vi "GD_Infos_Auswerten.vi"(11 "Sprachliste":string[][](array[string])) -> (1 "GD Info Text":string, 2 "GD Infos Array":string[](array[string]), 3 "GD Error occured":bool)   [LabVIEW 2020, in "Linearisierung v2.lvlib" / "SpanEinstellungen.lvlib"]
uses:
  SpanEinstellungen.lvlib
  Aktion FGV GD Errors sammeln.ctl
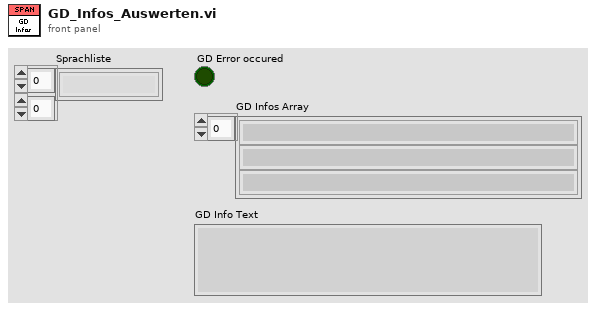
[diagram p1: front panel]
types:
  T1 = typedef "Linearisierung v2.lvlib/SpanEinstellungen.lvlib/Aktion FGV GD Errors sammeln.ctl" = enum16{"lesen", "init", "GD Infos sammeln", "Kalibrierinfos sammeln", "Test Data", "GD Infos selektiv sammeln"}
  T2 = typedef "Linearisierung v2.lvlib/SpanEinstellungen.lvlib/GD Info Cluster.ctl" = cluster{"Wobei":string, "Status":string, "Errors":T3, "Empfangsdaten":string[], "Zeitstempel":string}
  T3 = typedef "Linearisierung v2.lvlib/LIN ErrorCluster.ctl" = cluster{"Störung Kommunikation":bool, "Pressure carrier gas":bool, "Pressure diluted gas":bool, "Outlet Pressure":bool, "SNOX before SAIR":bool, "Störung Gasteiler":bool}
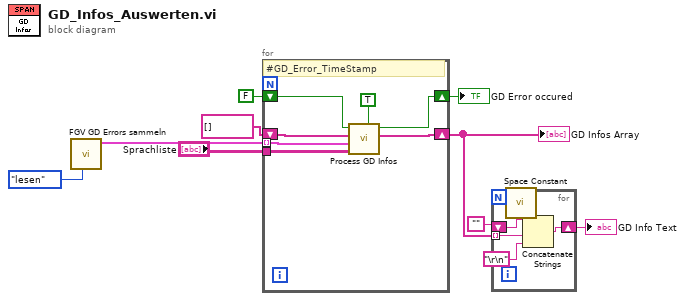
[diagram p0: block diagram]
diagram:
  n1 = call "FGV GD Errors sammeln.vi"("Aktion"=Aktion_FGV_GD_Errors_sammeln."lesen") -> ("GD Info-Cluster out"=w8:T2[])  [unwired: 8 in, 2 out]
  n2 = for {
    tunnel: w8 -> [w16] mode=indexing
    shift-right: [w15] -> w3
    shift-left: string[] [] -> [w12]
    shift-right: [w14] -> w5
    shift-left: FALSE -> [w13]
    tunnel: "Sprachliste" -> [w11]
    # "#GD_Error_TimeStamp"
    n3 = call "Process GD Infos.vi"("include Timestamp"=TRUE, "Sprachliste"=w11, "GD Info-Cluster in"=w16, "Array (Eingang)"=w12, "Error occured (Eingang)"=w13) -> ("Array (Ausgang)"=w15:string[], "Error occured (Ausgang)"=w14:bool)  [unwired: 4 in, 1 out]
  }
  "GD Infos Array" <- w3
  "GD Error occured" <- w5
  n4 = for {
    tunnel: w3 -> [w21] mode=indexing
    shift-right: [w20] -> w2
    shift-left: "" -> [w19]
    n5 = call <vilib>:"Space Constant.vi"() -> ("String"=w18:string)
    n6 = Concatenate Strings(w19, w18, w21, "\r\n") -> (w20:string)
  }
  "GD Info Text" <- w2
